vi "Ref_3_P.vi"(0 "Trip  Ch 1":refnum<vi>, 1 "Trip  Ch 2":refnum<vi>, 2 "Trip  Ch 11":refnum<vi>, 3 "Trip  Ch 3":refnum<vi>, 4 "Trip  Ch 4":refnum<vi>, 5 "Trip  Ch 5":refnum<vi>, 6 "Trip  Ch 12":refnum<vi>, 7 "Trip  Ch 6":refnum<vi>, 8 "Trip  Ch 7":refnum<vi>, 9 "Trip  Ch 8":refnum<vi>, 10 "Init_F":bool=TRUE, 12 "Trip  Ch 9":refnum<vi>, 13 "Trip  Ch 10":refnum<vi>) -> (14 "Trip  Ch 1 out":refnum<vi>, 15 "Trip  Ch 2 out":refnum<vi>, 16 "Trip  Ch 3 out":refnum<vi>, 17 "Trip  Ch 4 out":refnum<vi>, 19 "Trip  Ch 5 out":refnum<vi>, 20 "Trip  Ch 6 out":refnum<vi>, 21 "Trip  Ch 7 out":refnum<vi>, 22 "Trip  Ch 11 out":refnum<vi>, 23 "Trip  Ch 8 out":refnum<vi>, 24 "Trip  Ch 9 out":refnum<vi>, 25 "Trip  Ch 10 out":refnum<vi>, 26 "Trip  Ch 12 out":refnum<vi>)   [LabVIEW 2017]
panel:
  out "error out":errorcluster
  in  "error in":errorcluster
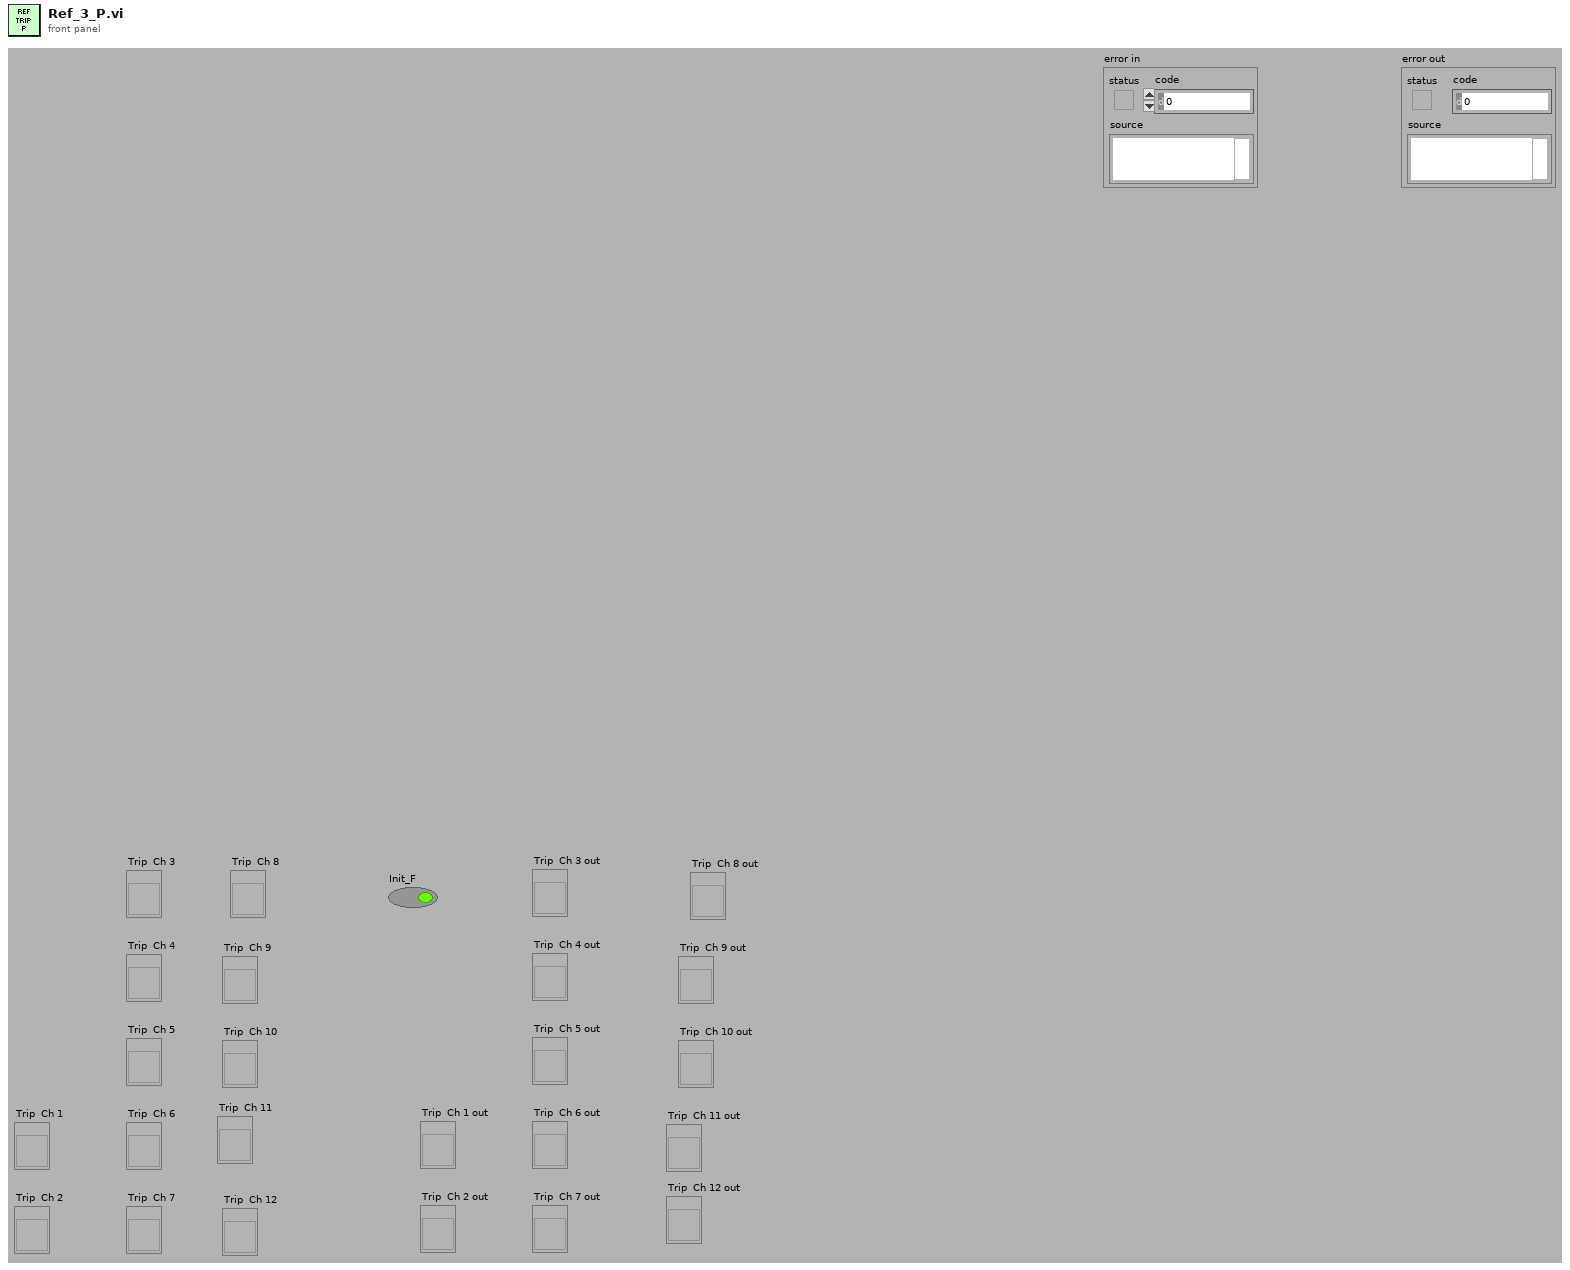
[diagram p1: front panel]
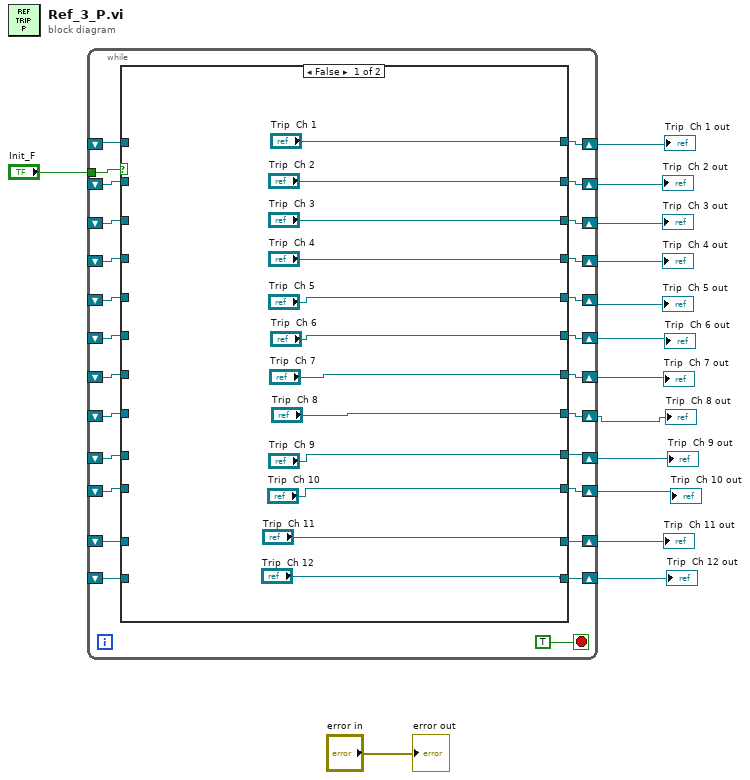
[diagram p0: block diagram]
diagram:
  n1 = while {
    shift-right: [w39] -> w6
    shift-left: _ -> [w38]
    tunnel: "Init_F" -> [w37]
    shift-right: [w36] -> w7
    shift-left: _ -> [w29]
    shift-right: [w35] -> w8
    shift-left: _ -> [w28]
    shift-right: [w34] -> w9
    shift-left: _ -> [w23]
    shift-right: [w33] -> w10
    shift-left: _ -> [w27]
    shift-right: [w32] -> w11
    shift-left: _ -> [w26]
    shift-right: [w31] -> w12
    shift-left: _ -> [w25]
    shift-right: [w30] -> w3
    shift-left: _ -> [w24]
    shift-right: [w22] -> w5
    shift-left: _ -> [w20]
    shift-right: [w21] -> w4
    shift-left: _ -> [w19]
    shift-right: [w18] -> w2
    shift-left: _ -> [w16]
    shift-right: [w17] -> w1
    shift-left: _ -> [w15]
    stop <- TRUE stop-if-true
    n2 = case shown="False" w37 {
      tunnel: ["Trip  Ch 1" w64] -> w39
      tunnel: w38 -> [_ w64]
      tunnel: ["Trip  Ch 2" w57] -> w36
      tunnel: ["Trip  Ch 3" w58] -> w35
      tunnel: ["Trip  Ch 4" w59] -> w34
      tunnel: ["Trip  Ch 5" w60] -> w33
      tunnel: ["Trip  Ch 6" w61] -> w32
      tunnel: ["Trip  Ch 7" w62] -> w31
      tunnel: ["Trip  Ch 8" w63] -> w30
      tunnel: w29 -> [_ w57]
      tunnel: w28 -> [_ w58]
      tunnel: w27 -> [_ w60]
      tunnel: w26 -> [_ w61]
      tunnel: w25 -> [_ w62]
      tunnel: w24 -> [_ w63]
      tunnel: w23 -> [_ w59]
      tunnel: ["Trip  Ch 9" w56] -> w22
      tunnel: ["Trip  Ch 10" w55] -> w21
      tunnel: w20 -> [_ w56]
      tunnel: w19 -> [_ w55]
      tunnel: ["Trip  Ch 11" w54] -> w18
      tunnel: ["Trip  Ch 12" w53] -> w17
      tunnel: w16 -> [_ w54]
      tunnel: w15 -> [_ w53]
      frame False {
      }
      frame True {
      }
    }
  }
  "Trip  Ch 8 out" <- w3
  "Trip  Ch 7 out" <- w12
  "Trip  Ch 6 out" <- w11
  "Trip  Ch 5 out" <- w10
  "Trip  Ch 4 out" <- w9
  "Trip  Ch 3 out" <- w8
  "Trip  Ch 2 out" <- w7
  "Trip  Ch 1 out" <- w6
  "Trip  Ch 9 out" <- w5
  "Trip  Ch 10 out" <- w4
  "Trip  Ch 11 out" <- w2
  "Trip  Ch 12 out" <- w1
  "error out" <- "error in"
